vi "Command Agitate Hopper.vi"(2 "Robot System Functions In":T1, 3 "Startup":bool, 4 "String Parameter":string, 5 "Cmd Parameter 3":dbl, 6 "Cmd Parameter 2":dbl, 7 "Cmd Parameter 1":dbl) -> (0 "Robot System Functions Out":T1, 1 "Completed":bool)   [LabVIEW 2016]
uses:
  Subsystems/All Robot Commands.ctl
  Subsystems/Drive and Climb SS/Drive + Climb Commands 2017.ctl
  Subsystems/Gear Delivery SS/Gear Delivery Commands.ctl
  Subsystems/Conveyor and Shooter SS/Conveyor and Shooter Commands.ctl
  Subsystems/Ball Intake SS/Ball Intake Commands.ctl
  Command Execution State.ctl
panel:
  # "Sample robot\ncontrol output.\nReplace with \nactual teleop \ncontrol signal \nstructure."
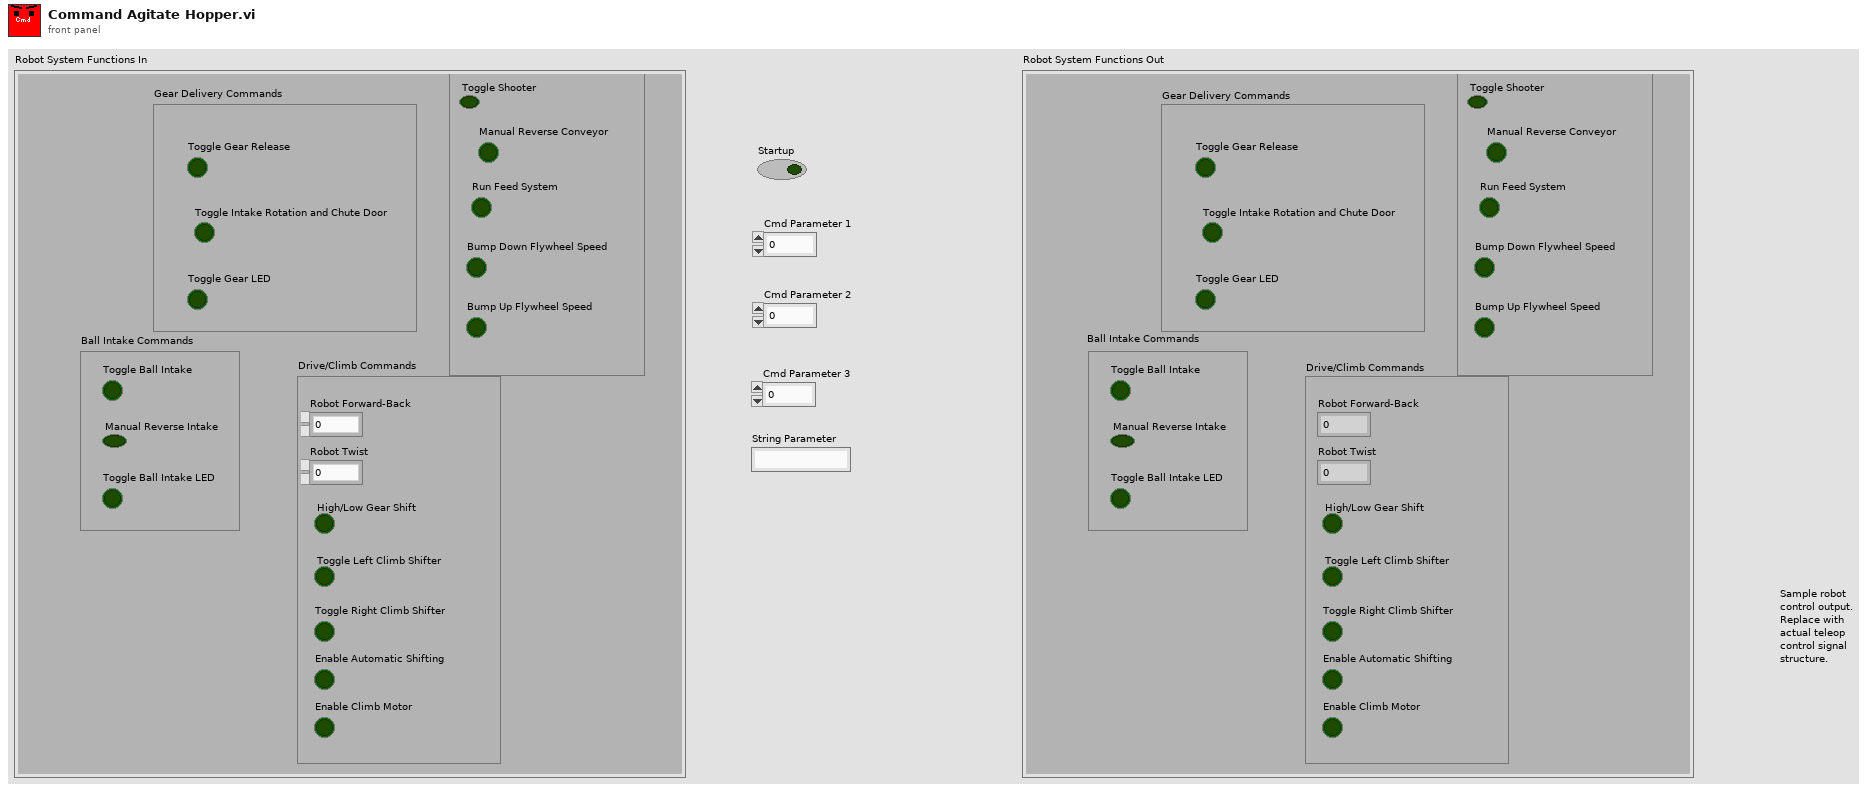
[diagram p1: front panel]
types:
  T1 = typedef "All Robot Commands.ctl" = cluster{"Drive/Climb Commands":T2, "Gear Delivery Commands":T3, "Shooter and Conveyor Commands":T4, "Ball Intake Commands":T5}
  T2 = typedef "Drive + Climb Commands 2017.ctl" = cluster{"Robot Forward-Back":dbl, "Robot Twist":dbl, "High/Low Gear Shift":bool, "Toggle Left Climb Shifter":bool, "Toggle Right Climb Shifter":bool, "Enable Automatic Shifting":bool, "Enable Climb Motor ":bool}
  T3 = typedef "Gear Delivery Commands.ctl" = cluster{"Toggle Gear Release":bool, "Toggle Intake Rotation and Chute Door":bool, "Toggle Gear LED":bool}
  T4 = typedef "Conveyor and Shooter Commands.ctl" = cluster{"Toggle Shooter":bool, "Manual Reverse Conveyor":bool, "Run Feed System":bool, "Bump Down Flywheel Speed":bool, "Bump Up Flywheel Speed":bool}
  T5 = typedef "Ball Intake Commands.ctl" = cluster{"Toggle Ball Intake":bool, "Manual Reverse Intake":bool, "Toggle Ball Intake LED":bool}
  T6 = typedef "Command Execution State.ctl" = enum16{"Initialize", "Execute", "Finish"}
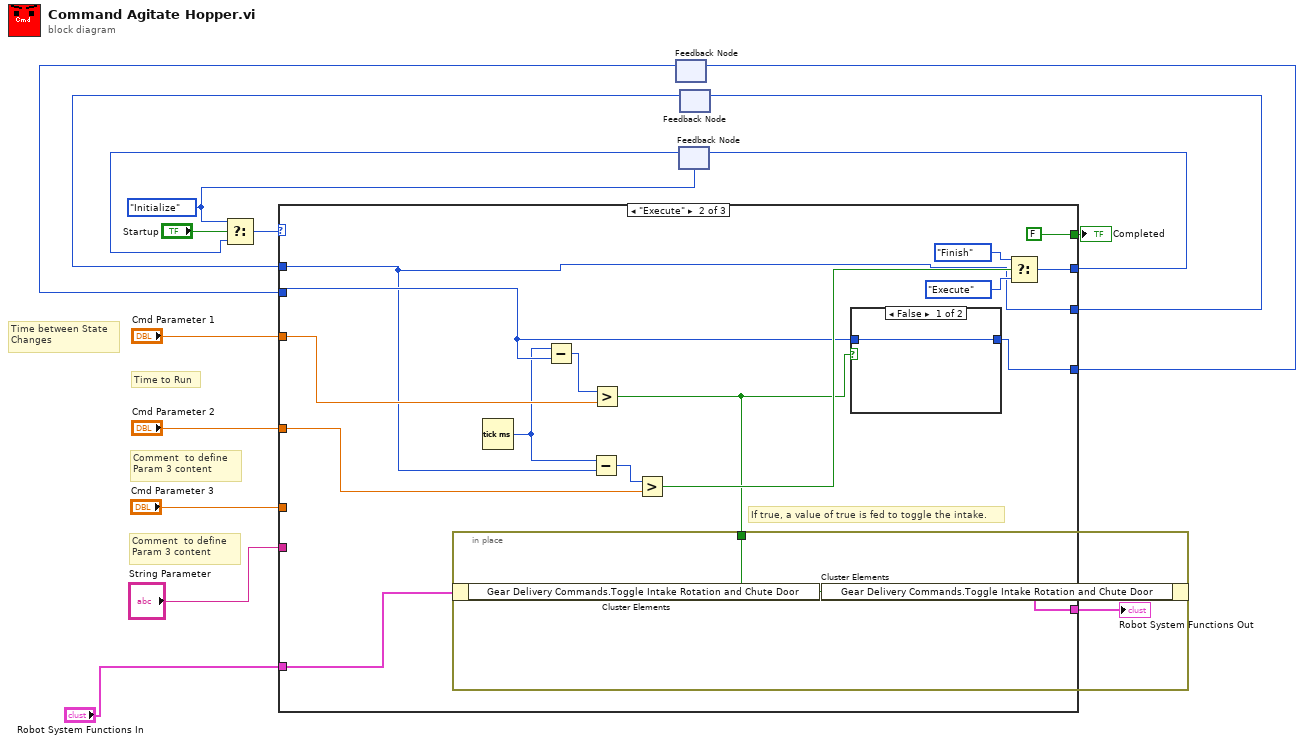
[diagram p0: block diagram]
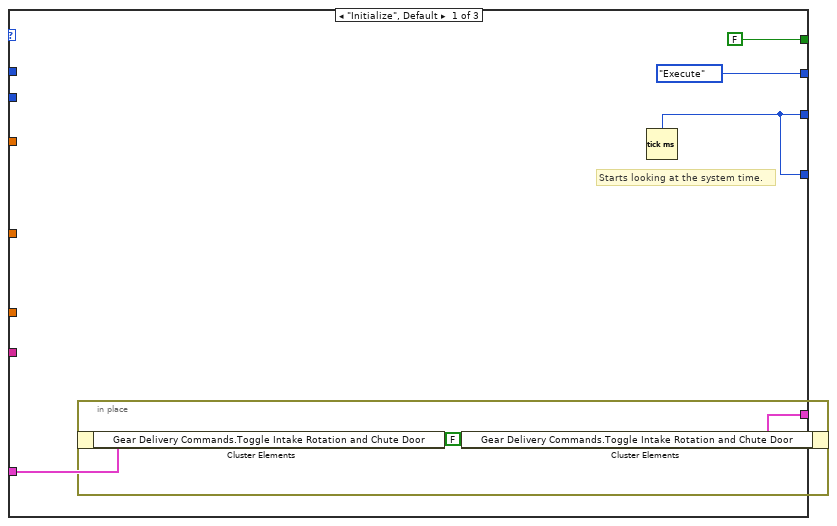
[diagram p2: hidden frame]
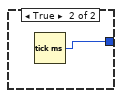
[diagram p3: hidden frame]
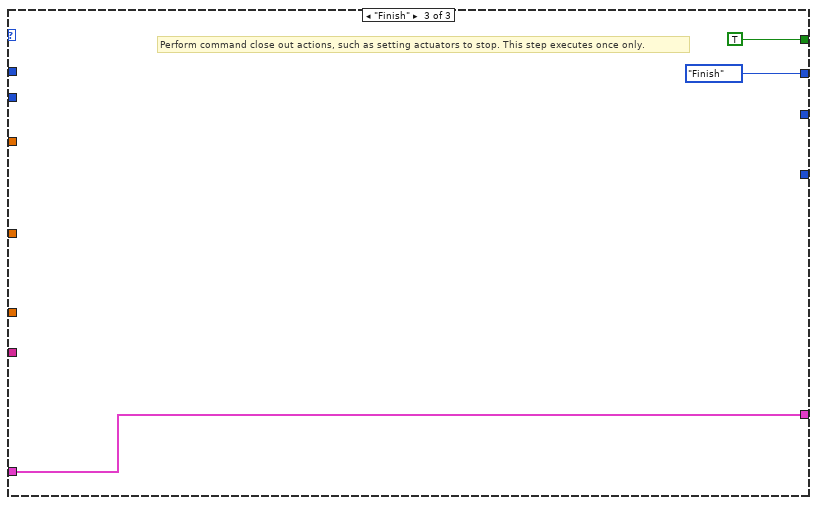
[diagram p4: hidden frame]
diagram:
  w11 = Command_Execution_State."Initialize" ("Play State")
  # "Comment  to define\nParam 3 content"
  # "Comment  to define\nParam 3 content"
  # "Time to Run"
  # "Time between State \nChanges"
  n1 = feedback #1() -> (w1:u32)  [unwired: 1 in]
  n2 = feedback #2(w11) -> (w12:T6)
  n3 = Select(t=w11, s="Startup", f=w12) -> (s? t:f=w16:T6)
  n4 = feedback #3() -> (w3:u32)  [unwired: 1 in]
  n5 = case shown="\"Execute\"" w16 {
    tunnel: [FALSE FALSE TRUE] -> w14
    tunnel: [Command_Execution_State."Execute" ("Play State") w36 Command_Execution_State."Finish" ("f")] -> w13
    tunnel: "Cmd Parameter 1" -> [_ w28 _]
    tunnel: "Cmd Parameter 2" -> [_ w25 _]
    tunnel: [w19 w32 w42] -> w8
    tunnel: "Robot System Functions In" -> [w18 w33 w42]
    tunnel: "Cmd Parameter 3" -> [_ _ _]
    tunnel: "String Parameter" -> [_ _ _]
    tunnel: [w17 w23 _] -> w4
    tunnel: w3 -> [_ w23 _]
    tunnel: [w17 w29 _] -> w2
    tunnel: w1 -> [_ w26 _]
    frame "Initialize", Default {
      # "Starts looking at the system time."
      n6 = in-place {
        n7 = in-place-cluster #4(w18) -> ()  [unwired: 1 out]
        n8 = in-place-cluster #4("Gear Delivery Commands.Toggle Intake Rotation and Chute Door"=FALSE ("Gear Delivery Commands.Toggle Intake Rotation")) -> (w19:T1)
      }
      n9 = Tick Count (ms)() -> (millisecond timer value=w17:u32)
    }
    frame "Execute" {
      # "If true, a value of true is fed to toggle the intake."
      n10 = Tick Count (ms)() -> (millisecond timer value=w24:u32)
      n11 = Subtract(x=w24, y=w26) -> (x-y=w27:u32)
      n12 = Subtract(x=w24, y=w23) -> (x-y=w31:u32)
      n13 = Greater?(x=w27, y=w28) -> (0:w30:bool)
      n14 = in-place {
        in-place-border: w30 -> [w41]
        n15 = in-place-cluster #5(w33) -> ()  [unwired: 1 out]
        n16 = in-place-cluster #5("Gear Delivery Commands.Toggle Intake Rotation and Chute Door"=w41) -> (w32:T1)
      }
      n17 = Greater?(x=w31, y=w25) -> (0:w34:bool)
      n18 = case shown="False" w30 {
        tunnel: [w39 w40] -> w29
        tunnel: w26 -> [w39 _]
        frame False {
        }
        frame True {
          n19 = Tick Count (ms)() -> (millisecond timer value=w40:u32)
        }
      }
      n20 = Select(t=Command_Execution_State."Finish" ("Play State"), s=w34, f=Command_Execution_State."Execute") -> (s? t:f=w36:T6)
    }
    frame "Finish" {
      # "Perform command close out actions, such as setting actuators to stop. This step executes once only."
    }
  }
  "Completed" <- w14
  "Robot System Functions Out" <- w8
  n21 = feedback-in #1(w2) -> ()
  n22 = feedback-in #2(w13) -> ()
  n23 = feedback-in #3(w4) -> ()
